vi "20170502-lecture4-1 write to file txt.vi"   [LabVIEW 2014]
types:
  T1 = enum16{"open", "replace", "create", "open or create", "replace or create", "replace or create with confirmation"}
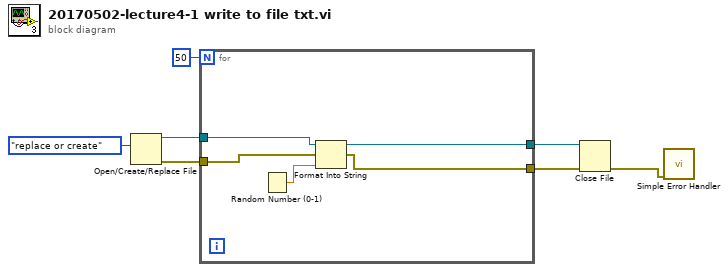
[diagram p0: block diagram]
diagram:
  n1 = Open/Create/Replace File(operation (0:open)=T1."replace or create") -> (refnum out=w5:refnum<file>, error out=w4:errorcluster)  [unwired: 5 in, 1 out]
  n2 = for {
    N: 50 -> [_]
    tunnel: w5 -> [w11]
    tunnel: w4 -> [w10]
    tunnel: [w9] -> w3
    tunnel: [w8] -> w2
    n3 = Random Number (0-1)() -> (number: 0 to 1=w12:dbl)
    n4 = Format Into String(initial string=w11, error in=w10, w12) -> (resulting string=w9:refnum<file>, error out=w8:errorcluster)  [unwired: 1 in]
  }
  n5 = Close File(refnum=w3, error in=w2) -> (error out=w1:errorcluster)  [unwired: 1 out]
  n6 = call <vilib>:"Simple Error Handler.vi"("error in (no error)"=w1) -> ()  [unwired: 4 in, 5 out]
